vi "file error to exception.vi"(8 "exception in":T1 {"code" format="%.0x"}, 10 "file path":path, 11 "error in":errorcluster) -> (0 "exception":T1 {"code" format="%.0x"})   [LabVIEW 2013, in "file errors.lvlib"]
uses:
  file errors.lvlib
  exception.lvlib
  exception.ctl
  Variant Repository/Write Variant Repository/Write Exception Property.xnode
  <vilib>/Utility/VariantDataType/GetTypeInfo.vi
  <vilib>/Utility/VariantDataType/VariantType.lvlib
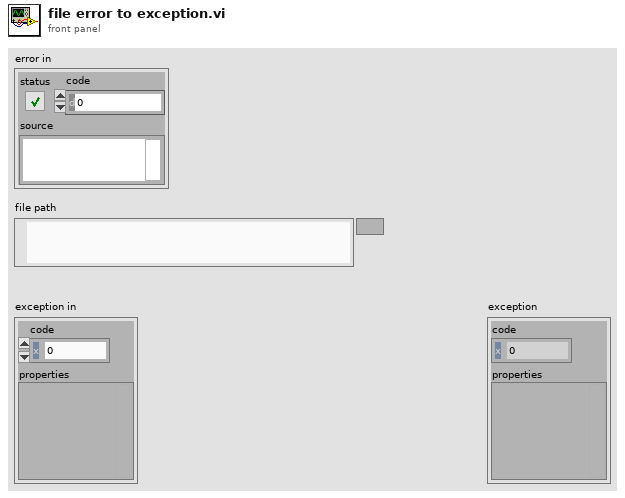
[diagram p1: front panel]
types:
  T1 = typedef "exception.lvlib/exception.ctl" = cluster{"code":i32, "properties":variant}
  T2 = typedef "exception.lvlib/severity.ctl" = enum8{"unspecified", "informational", "operation failed", "data corruption", "system corruption", "critical unknown state"}
  T3 = typedef "file errors.lvlib/file error.ctl" = enum16{"invalid path or reference", "end of file", "file already opened", "generic file error", "file not found", "permissions invalid", "disk full", "duplicate path", "too many open file handles", "useless generic error"}
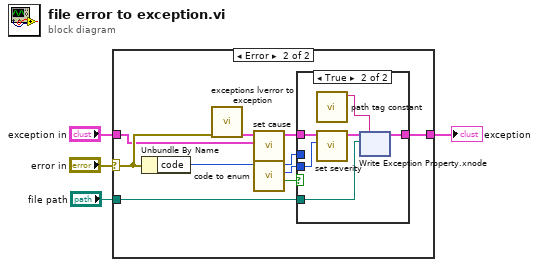
[diagram p0: block diagram]
diagram:
  n1 = case shown="Error" "error in" {
    selector: "error in" -> [_ w9]
    tunnel: "exception in" -> [w5 w7]
    tunnel: [w5 w15] -> w3
    tunnel: "file path" -> [_ w14]
    frame No Error {
    }
    frame Error {
      n2 = Unbundle By Name(w9) -> ("code"=w13:i32)
      n3 = call "exceptions lverror to exception.vi"("error in"=w9) -> ("exception"=w8:T1)  [unwired: 10 in]
      n4 = call "set cause.vi"("cause"=w7, "exception in"=w8) -> ("exception out"=w6:T1)  [unwired: 9 in]
      n5 = call "code to enum.vi"("code"=w13) -> ("valid?"=w12:bool, "severity"=w11:T2, "file error"=w10:T3)  [unwired: 8 in]
      n6 = case shown="True" w12 {
        tunnel: w6 -> [w16 w18]
        tunnel: [w16 w17] -> w15
        tunnel: w14 -> [_ w19]
        tunnel: w11 -> [_ w21]
        tunnel: w10 -> [_ _]
        frame False {
        }
        frame True {
          n7 = call "path tag constant.vi"() -> ("Tag"=w22:string)  [unwired: 11 in]
          n8 = call "set severity.vi"("severity"=w21, "exception in"=w18) -> ("exception out"=w20:T1)  [unwired: 9 in]
          n9 = xnode "Write Exception Property.xnode"("exception in"=w20, "Tag"=w22, "Value"=w19) -> ("exception out"=w17:T1)  [unwired: 1 out]
        }
      }
    }
  }
  "exception" <- w3
